vi "CRYRead from Sequence to Tree Icon.vi"(8 "Is Refresh?":bool, 11 "StepsRef in":refnum<vi>) -> (0 "error out":errorcluster, 3 "StepsRefOut":refnum<vi>)   [LabVIEW 2013]
uses:
  CRYMainGlobal.vi
panel:
  in  "Sequences":string(tree)
  in  "Tags":string[](array[string])
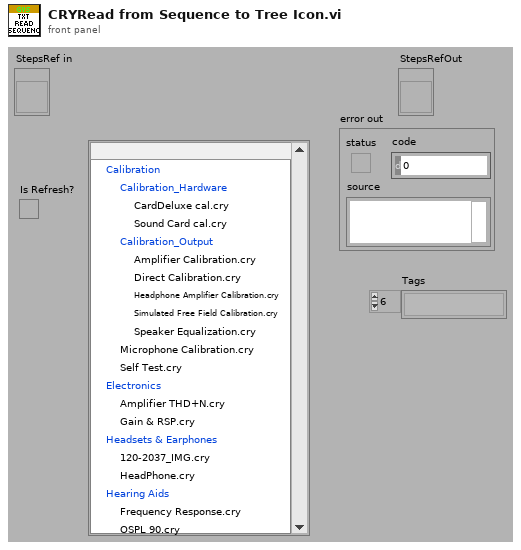
[diagram p1: front panel]
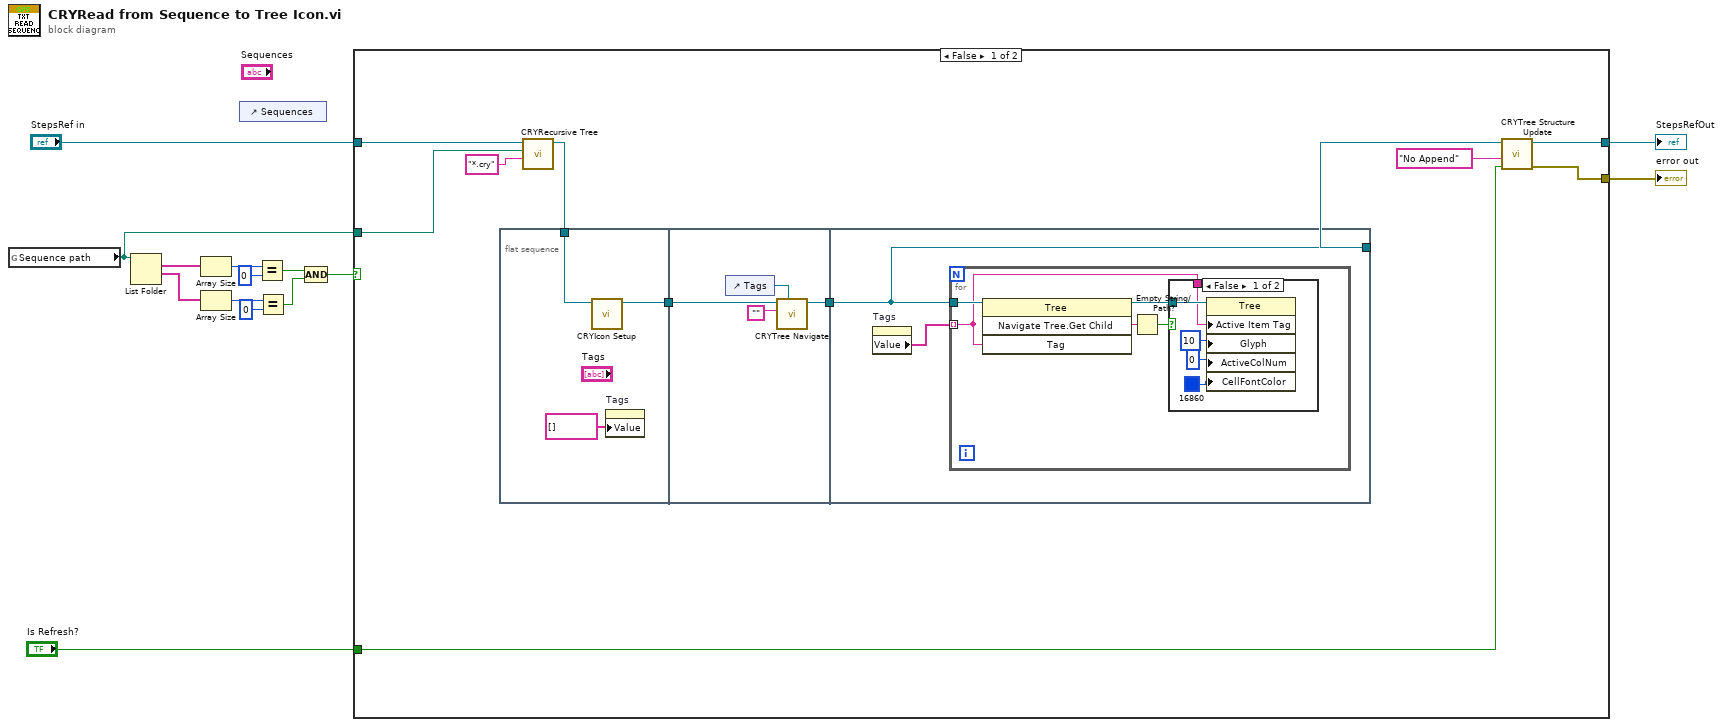
[diagram p0: block diagram]
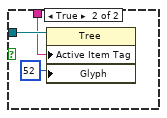
[diagram p2: hidden frame]
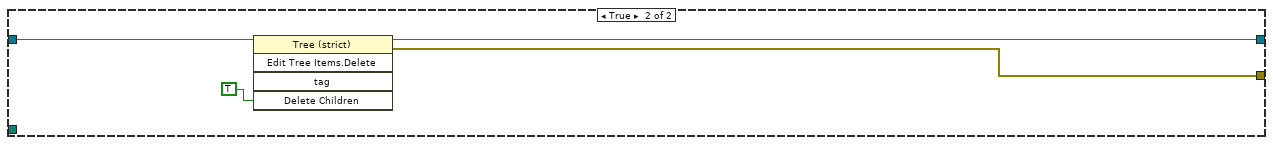
[diagram p3: hidden frame]
diagram:
  n1 = global read "CRYMainGlobal.vi" "Sequence path"() -> (w2:path)
  n2 = List Folder(path=w2) -> (filenames=w10:string[], folder names=w5:string[])  [unwired: 1 in, 4 out]
  n3 = Array Size(array=w10) -> (size(s)=w12:i32)
  n4 = Array Size(array=w5) -> (size(s)=w6:i32)
  n5 = control-ref of="Sequences"() -> ()  [unwired: 1 out]
  n6 = Equal?(x=w12, y=0) -> (x = y?=w9:bool)
  n7 = Equal?(x=w6, y=0) -> (x = y?=w3:bool)
  n8 = Compound Arithmetic op=AND(w9, w3) -> (w4:bool)
  n9 = case shown="False" w4 {
    tunnel: [w24 w49] -> w14
    tunnel: "StepsRef in" -> [w22 w50]
    tunnel: [w23 w48] -> w13
    tunnel: "Is Refresh?" -> [w25 _]
    tunnel: w2 -> [w21 _]
    frame False {
      n10 = flat-sequence {
        tunnel: w17 -> [w27]
        tunnel: [w26] -> w16
        tunnel: [w30] -> w19
        tunnel: w16 -> [w29]
        tunnel: w19 -> [w33]
        tunnel: [w33] -> w18
        frame #0 {
          n11 = call "CRYIcon Setup.vi"("TS Tree In"=w27) -> ("Tree ref"=w26:refnum<vi>)  [unwired: 1 in, 7 out]
          n12 = property on="Tags" class="Arr (strict)"("Value"=string[] [] ("Tags")) -> ()  [unwired: 2 in, 2 out]
        }
        frame #1 {
          n13 = control-ref of="Tags"() -> (w32:refnum<vi>)
          n14 = call "CRYTree Navigate.vi"("Tags"=w32, "Start Tag In"="", "Tree In"=w29) -> ("Tree Out"=w30:refnum<vi>)  [unwired: 8 in]
        }
        frame #2 {
          n15 = property on="Tags" class="Arr (strict)"() -> ("Value"=w34:string[])  [unwired: 2 in, 2 out]
          n16 = for {
            tunnel: w33 -> [w39]
            tunnel: w34 -> [w38] mode=indexing
            n17 = invoke class="Tree" method="Navigate Tree.Get Child"(reference=w39, "Tag"=w38) -> (reference out=w37:refnum<vi>, "Navigate Tree:Get Child"=w36:string)  [unwired: 2 in, 2 out]
            n18 = Empty String/Path?(string/path=w36) -> (empty?=w35:bool)
            n19 = case shown="False" w35 {
              tunnel: w37 -> [w44 w47]
              tunnel: w38 -> [w43 w46]
              frame False {
                n20 = property class="Tree"(reference=w44, "Active Item Tag"=w43, "Glyph"=10 ("Active Item:Symbol Index"), "ActiveColNum"=0 ("Active Cell:Active Column Number"), "CellFontColor"=u32 16860) -> ()  [unwired: 1 in, 2 out]
              }
              frame True {
                n21 = property class="Tree"(reference=w47, "Active Item Tag"=w46, "Glyph"=52 ("Active Item:Symbol Index")) -> ()  [unwired: 1 in, 2 out]
              }
            }
          }
        }
      }
      n22 = call "CRYRecursive Tree.vi"("pattern"="*.cry", "Sequence path"=w21, "Tree in"=w22) -> ("Tree Out"=w17:refnum<vi>)  [unwired: 8 in]
      n23 = call "CRYTree Structure Update.vi"("Is Refresh?"=w25, "Option"="No Append", "StepsRef in"=w18) -> ("error out"=w23:errorcluster, "StepsRefOut"=w24:refnum<vi>)  [unwired: 7 in]
    }
    frame True {
      n24 = invoke class="Tree (strict)" method="Edit Tree Items.Delete"(reference=w50, "Delete Children"=TRUE ("Delete Children?")) -> (reference out=w49:refnum<vi>, error out=w48:errorcluster)  [unwired: 3 in, 3 out]
    }
  }
  "StepsRefOut" <- w14
  "error out" <- w13
